vi "UpdateSaveRootPath.vi"(8 "error in (no error)":errorcluster, 11 "Scan Data Process in":T1) -> (0 "error out":errorcluster, 3 "Scan Data Process out":T1)   [LabVIEW 2015, in "Exposure Process.lvlib"]
uses:
  Exposure Process.lvlib
  Control_Scan Data Process.ctl
  <vilib>/addons/PointValueMap/controls/PointMap.ctl
  Control_EXP Information.ctl
  Control_File Save Setup.ctl
  Control_Enable and Path.ctl
  Control_ICM Export Setting.ctl
  ConfigHelper/ConfigHelper.lvlib
  <vilib>/addons/PointValueMap/PointValueMap.lvlib
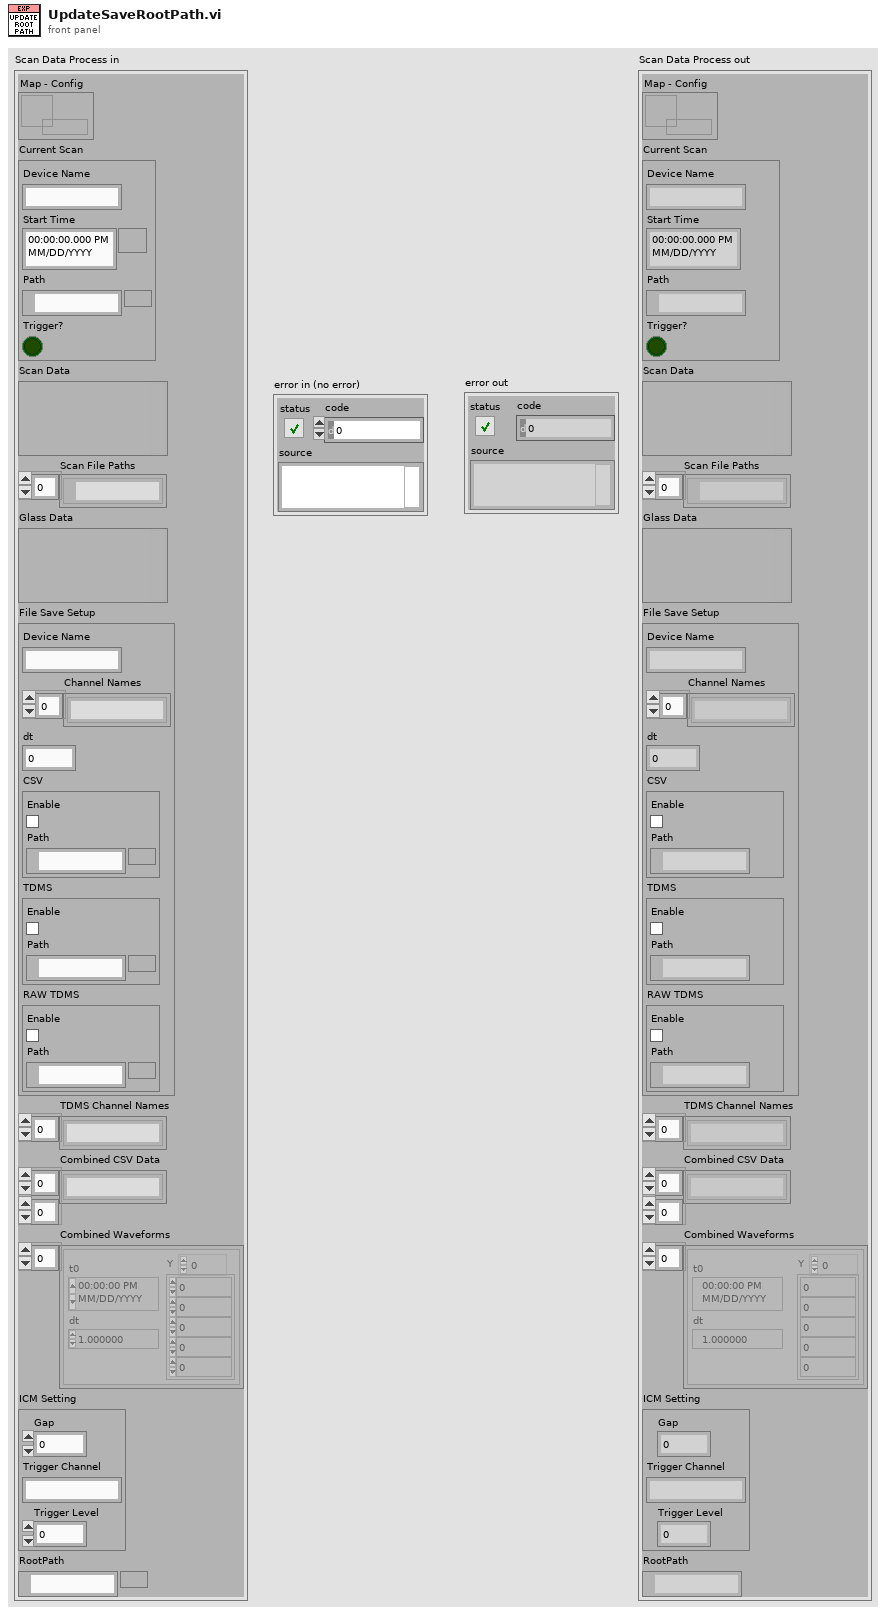
[diagram p1: front panel]
types:
  T1 = typedef "Exposure Process.lvlib/Control_Scan Data Process.ctl" = cluster{"Map - Config":T2, "Current Scan":T3, "Scan Data":variant, "Scan File Paths":path[], "Glass Data":variant, "File Save Setup":T4, "TDMS Channel Names":string[], "Combined CSV Data":string[][], "Combined Waveforms":waveform(dbl)[], "ICM Setting":T6, "RootPath":path}
  T2 = typedef "PointValueMap.lvlib/PointMap.ctl" = refnum<data-value>
  T3 = typedef "Exposure Process.lvlib/Control_EXP Information.ctl" = cluster{"Device Name":string, "Start Time":timestamp, "Path":path, "Trigger?":bool}
  T4 = typedef "Exposure Process.lvlib/Control_File Save Setup.ctl" = cluster{"Device Name":string, "Channel Names":string[], "dt":dbl, "CSV":T5, "TDMS":T5, "RAW TDMS":T5}
  T5 = typedef "Exposure Process.lvlib/Control_Enable and Path.ctl" = cluster{"Enable":bool, "Path":path}
  T6 = typedef "Exposure Process.lvlib/Control_ICM Export Setting.ctl" = cluster{"Gap":dbl, "Trigger Channel":string, "Trigger Level":dbl}
  T7 = typedef "ConfigHelper.lvlib/Config.ctl" = cluster{"Path":string, "Days to Keep":i32, "Number of Rows":i32}
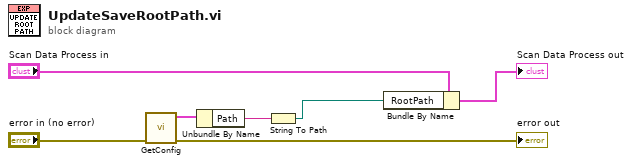
[diagram p0: block diagram]
diagram:
  n1 = call "GetConfig.vi"("error in (no error)"="error in (no error)") -> ("error out"=→"error out":errorcluster, "Config"=w4:T7)  [unwired: 9 in]
  n2 = Unbundle By Name(w4) -> ("Path"=w3:string)
  n3 = String To Path(string=w3) -> (path=w2:path)
  n4 = Bundle By Name(cluster="Scan Data Process in", "RootPath"=w2) -> (→"Scan Data Process out":T1)
